vi "Log Data.vi"(6 "error in (no error)":errorcluster, 7 "Logging Configuration":T3, 10 "Data w Time":T1, 11 "Calibration Configuration":T2) -> (4 "error out":errorcluster)   [LabVIEW 2024]
doc: "Use the Write To Measurement File Express VI to log data to disk in a LVM file."
uses:
  Logging Configuration.ctl
  Configuration/Calibration Configuration.ctl
  support/Control/Data Constant.ctl
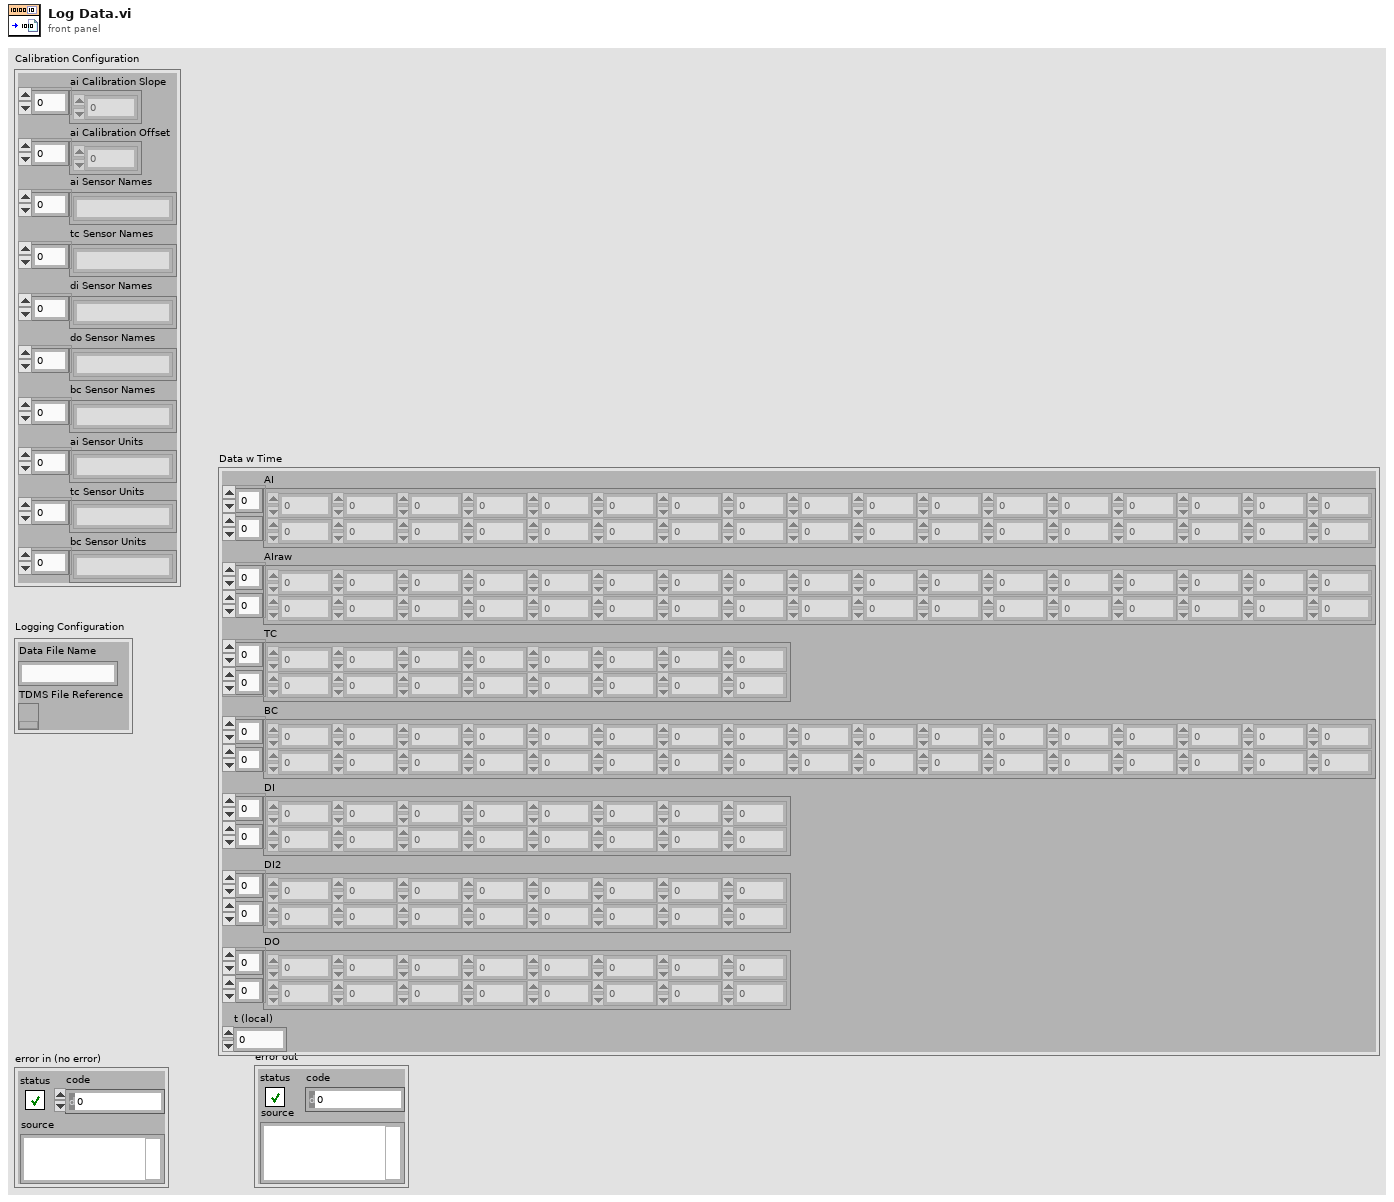
[diagram p1: front panel]
types:
  T1 = typedef "Data Constant.ctl" = cluster{"AI":dbl[][], "AIraw":dbl[][], "TC":dbl[][], "BC":dbl[][], "DI":dbl[][], "DI2":dbl[][], "DO":dbl[][], "t (local)":dbl}
  T2 = typedef "Calibration Configuration.ctl" = cluster{"ai Calibration Slope":dbl[], "ai Calibration Offset":dbl[], "ai Sensor Names ":string[], "tc Sensor Names":string[], "di Sensor Names":string[], "do Sensor Names":string[], "bc Sensor Names":string[], "ai Sensor Units":string[], "tc Sensor Units":string[], "bc Sensor Units":string[]}
  T3 = typedef "Logging Configuration.ctl" = cluster{"Data File Name":string, "TDMS File Reference":refnum<k34>}
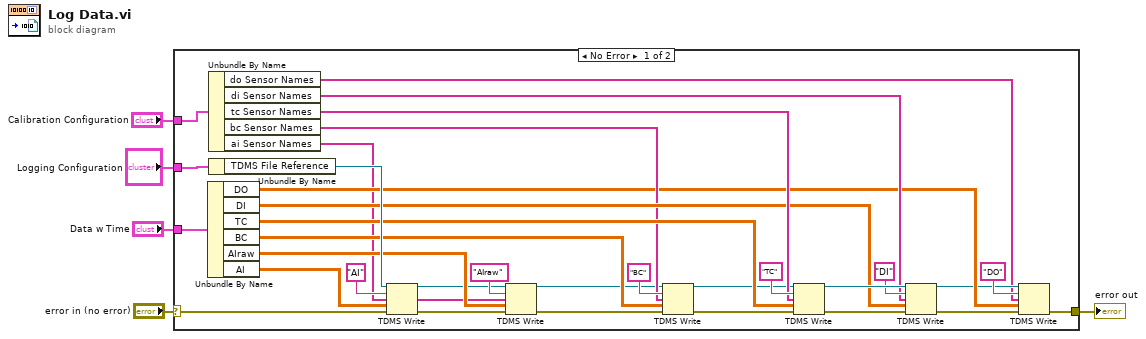
[diagram p0: block diagram]
diagram:
  n1 = case shown="No Error" "error in (no error)" {
    selector: "error in (no error)" -> [w37 w39]
    tunnel: "Logging Configuration" -> [w38 _]
    tunnel: [w17 w39] -> w4
    tunnel: "Calibration Configuration" -> [w33 _]
    tunnel: "Data w Time" -> [w31 _]
    frame No Error {
      n2 = Unbundle By Name(w31) -> ("DO"=w16:dbl[][], "DI"=w27:dbl[][], "TC"=w30:dbl[][], "BC"=w22:dbl[][], "AIraw"=w11:dbl[][], "AI"=w12:dbl[][])
      n3 = Unbundle By Name(w33) -> ("do Sensor Names"=w14:string[], "di Sensor Names"=w25:string[], "tc Sensor Names"=w32:string[], "bc Sensor Names"=w20:string[], "ai Sensor Names"=w6:string[])
      n4 = Unbundle By Name(w38) -> ("TDMS File Reference"=w36:refnum<k34>)
      n5 = TDMS Write(0:w36, 5:"AI", 7:w6, 9:w12, 11:w37) -> (4:w7:refnum<k34>, 15:w9:errorcluster)  [unwired: 1 in, 2 out]
      n6 = TDMS Write(0:w7, 5:"AIraw" ("group name in (Untitled)"), 7:w6, 9:w11, 11:w9) -> (4:w8:refnum<k34>, 15:w10:errorcluster)  [unwired: 1 in, 2 out]
      n7 = TDMS Write(0:w8, 5:"BC" ("group name in (Untitled)"), 7:w20, 9:w22, 11:w10) -> (4:w23:refnum<k34>, 15:w24:errorcluster)  [unwired: 1 in, 2 out]
      n8 = TDMS Write(0:w23, 5:"TC", 7:w32, 9:w30, 11:w24) -> (4:w28:refnum<k34>, 15:w29:errorcluster)  [unwired: 1 in, 2 out]
      n9 = TDMS Write(0:w28, 5:"DI", 7:w25, 9:w27, 11:w29) -> (4:w15:refnum<k34>, 15:w18:errorcluster)  [unwired: 1 in, 2 out]
      n10 = TDMS Write(0:w15, 5:"DO", 7:w14, 9:w16, 11:w18) -> (15:w17:errorcluster)  [unwired: 1 in, 3 out]
    }
    frame Error {
    }
  }
  "error out" <- w4
